vi "GetStageParam.vi"(8 "error in (no error)":errorcluster, 10 "StageParamInput":T1[](array[typedef]), 11 "vi reference":refnum<vi>) -> (0 "error out":errorcluster, 2 "StageParamOutput":T1[](array[typedef]), 3 "vi ref out":refnum<vi>)   [LabVIEW 2017]
doc: "Use this template to build a VI to use as a subVI."
uses:
  Utility/AxisControl.ctl
  SingleStageData.ctl
panel:
  in  "Execute":bool
  in  "Distance":dbl
  in  "Jog Left":bool
  out "Pos Fbk":dbl
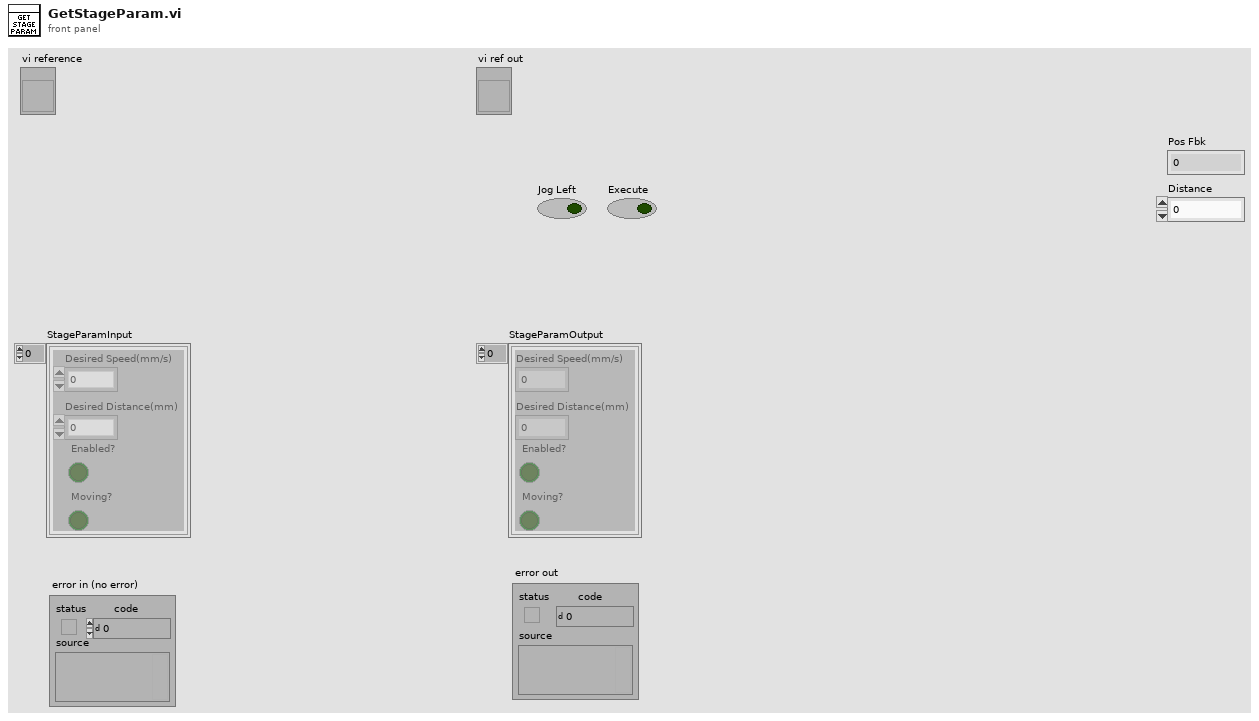
[diagram p1: front panel]
types:
  T1 = typedef "SingleStageData.ctl" = cluster{"Desired Speed(mm/s)":dbl, "Desired Distance(mm)":dbl, "Enabled?":bool, "Moving?":bool}
  T2 = typedef "AxisControl.ctl" = cluster{"Axis":string, "Enable":bool, "Disable":bool, "Home":bool, "FaultAck":bool, "Jog":bool, "Speed":dbl, "Distance":dbl, "Jog Left":bool, "Jog Right":bool, "Status":string, "Pos Fbk":dbl, "Vel Fbk":dbl, "Pos Units":string, "Vel Units":string}
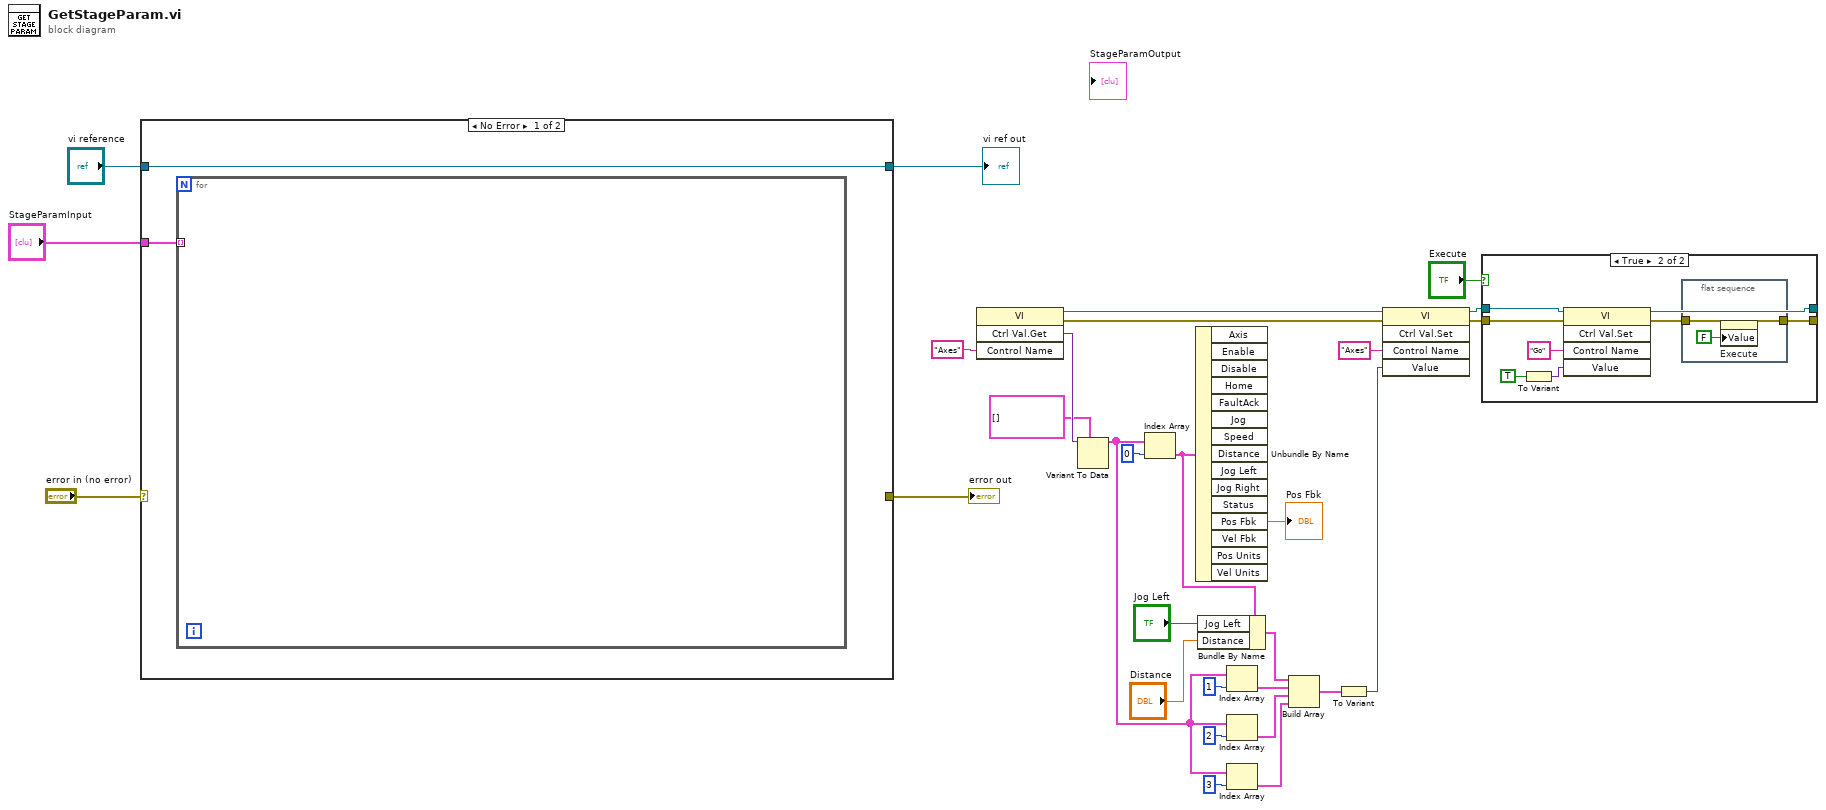
[diagram p0: block diagram]
diagram:
  n1 = case shown="No Error" "error in (no error)" {
    selector: "error in (no error)" -> [_ w35]
    tunnel: [_ w35] -> w30
    tunnel: [w33 w34] -> w29
    tunnel: "vi reference" -> [w33 w34]
    tunnel: "StageParamInput" -> [w32 _]
    frame No Error {
      n2 = for {
        tunnel: w32 -> [_] mode=indexing
      }
    }
    frame Error {
    }
  }
  "error out" <- w30
  "vi ref out" <- w29
  n3 = invoke class="VI" method="Ctrl Val.Get"("Control Name"="Axes") -> (reference=w26:refnum<vi>, reference out=w19:refnum<vi>, error in=w25:errorcluster, error out=w18:errorcluster, "Get Control Value Variant"=w23:variant)  [unwired: 1 in, 1 out]
  n4 = Variant To Data(type=T2[] [], Variant=w23) -> (data=w7:T2[])  [unwired: 1 in, 1 out]
  n5 = Index Array(array=w7, index=0) -> (element=w16:T2)
  n6 = Unbundle By Name(w16) -> ("Pos Fbk"=→"Pos Fbk":dbl)  [unwired: 14 out]
  n7 = Bundle By Name(cluster=w16, "Jog Left"="Jog Left", "Distance"="Distance") -> (w15:T2)
  n8 = Index Array(array=w7, index=1) -> (element=w13:T2)
  n9 = Index Array(array=w7, index=2) -> (element=w6:T2)
  n10 = Index Array(array=w7, index=3) -> (element=w5:T2)
  n11 = Build Array(w15, w13, w6, w5) -> (w12:T2[])
  n12 = To Variant(anything=w12) -> (Variant=w11:variant)
  n13 = invoke class="VI" method="Ctrl Val.Set"(reference=w19, error in=w18, "Control Name"="Axes", "Value"=w11) -> (reference out=w1:refnum<vi>, error out=w2:errorcluster)  [unwired: 1 in, 3 out]
  n14 = case shown="True" "Execute" {
    tunnel: w1 -> [w36 w45]
    tunnel: w2 -> [w37 w44]
    tunnel: [w37 w38] -> _
    tunnel: [w36 w43] -> _
    frame False {
    }
    frame True {
      n15 = To Variant(anything=TRUE) -> (Variant=w41:variant)
      n16 = invoke class="VI" method="Ctrl Val.Set"(reference=w45, error in=w44, "Control Name"="Go", "Value"=w41) -> (reference out=w43:refnum<vi>, error out=w39:errorcluster)  [unwired: 1 in, 3 out]
      n17 = flat-sequence {
        tunnel: w39 -> [w47]
        tunnel: [w47] -> w38
        frame #0 {
          n18 = property on="Execute" class="Bool (strict)"("Value"=FALSE ("Execute")) -> ()  [unwired: 2 in, 2 out]
        }
      }
    }
  }
